vi "Write Text.vi"(5 "Text":refnum<class "Text.lvclass">, 9 "String in":refnum<class "String.lvclass">) -> (3 "String out":refnum<class "String.lvclass">)   [LabVIEW 2014, in "String.lvclass"]
uses:
  String.lvclass
  Text/Text.lvclass
  String.lvclass/String.ctl
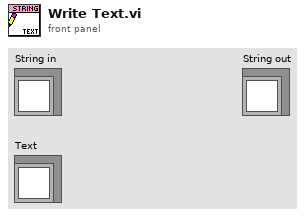
[diagram p1: front panel]
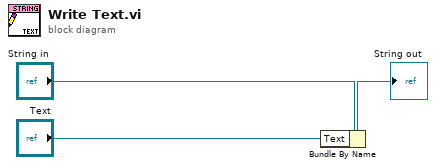
[diagram p0: block diagram]
diagram:
  n1 = Bundle By Name(cluster="String in", "Text"="Text") -> (→"String out":refnum<class "String.lvclass">)
